vi "Ring_buffer_reader_Core.vi"() -> ()   [LabVIEW 2011]
panel:
  out "Array 2":T1(array[cluster])
  in  "Array":path[](array[path])=[path "C:/Franjo/Work/2014/CoDiS_Core/CoDiS-DM_PS_Wivenhoe/Temp/Running_Log_7/CPU_Usage (%).bin"]
  out "Remainder2":i64
  out "Loop Count 2":i32
  out "Remainder1":i64
  out "size (in bytes)":i64
  out "Loop Count 1":i32
  out "pointer":i64
  out "XY Graph":T1(graph)
  out "error out":errorcluster
  # "03:02:50"
  # "Remainder1 and Remainder2 should be zero, otherwise file is corrupted."
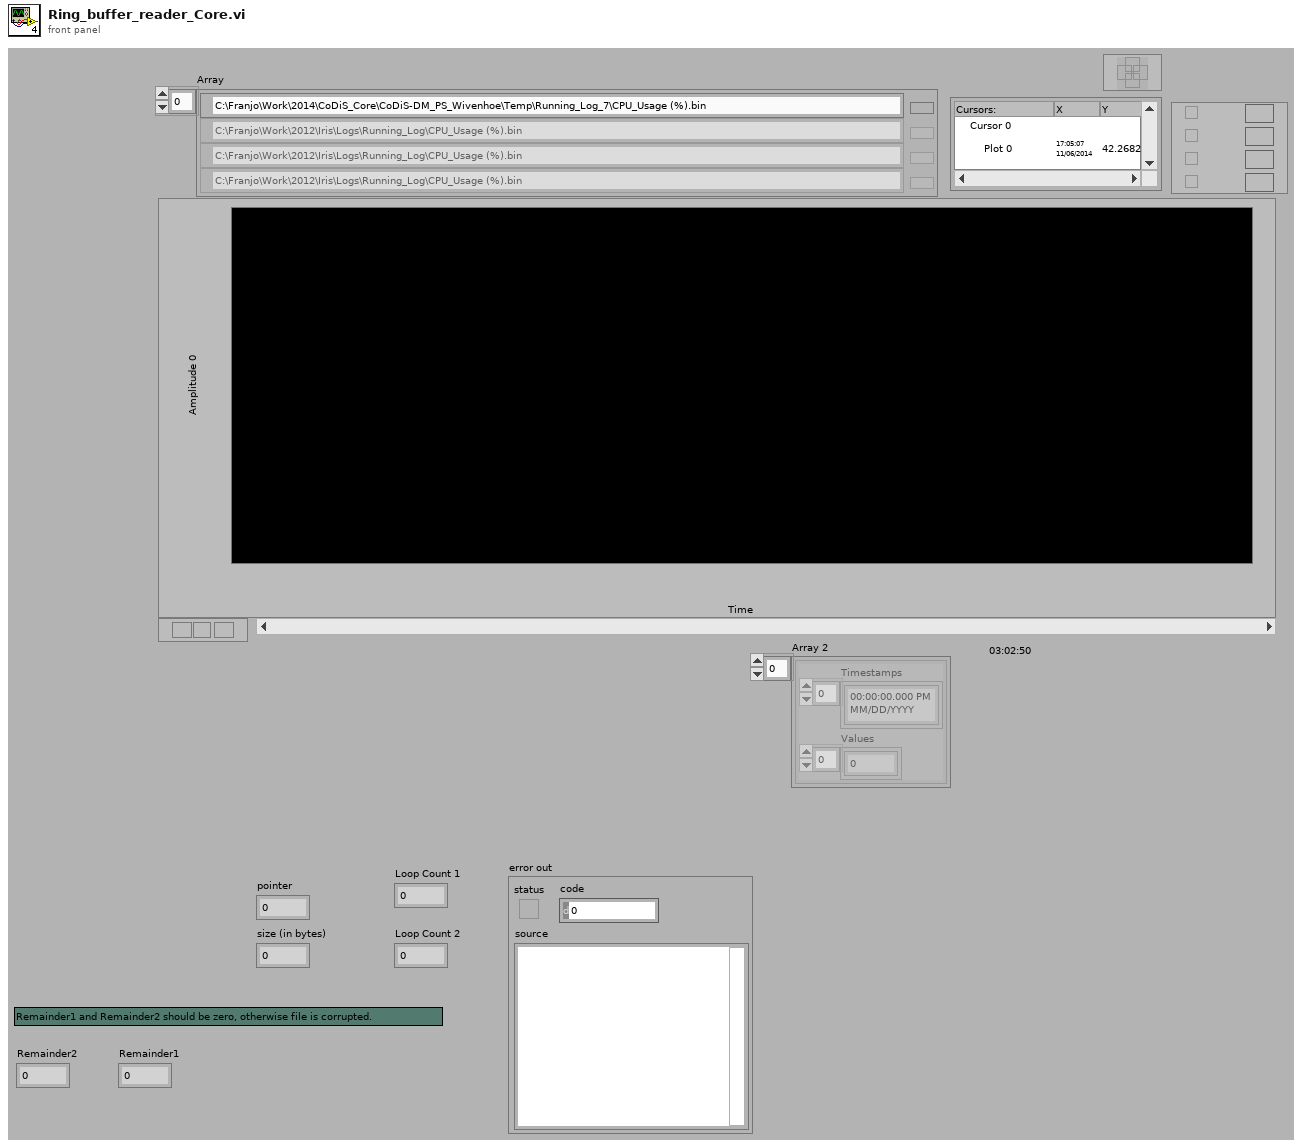
[diagram p1: front panel]
types:
  T1 = cluster{"Timestamps":timestamp[], "Values":sgl[]}[]
  T2 = cluster{"Timestamps":timestamp[], "Values":sgl[]}
  T3 = enum16{"open", "replace", "create", "open or create", "replace or create", "replace or create with confirmation"}
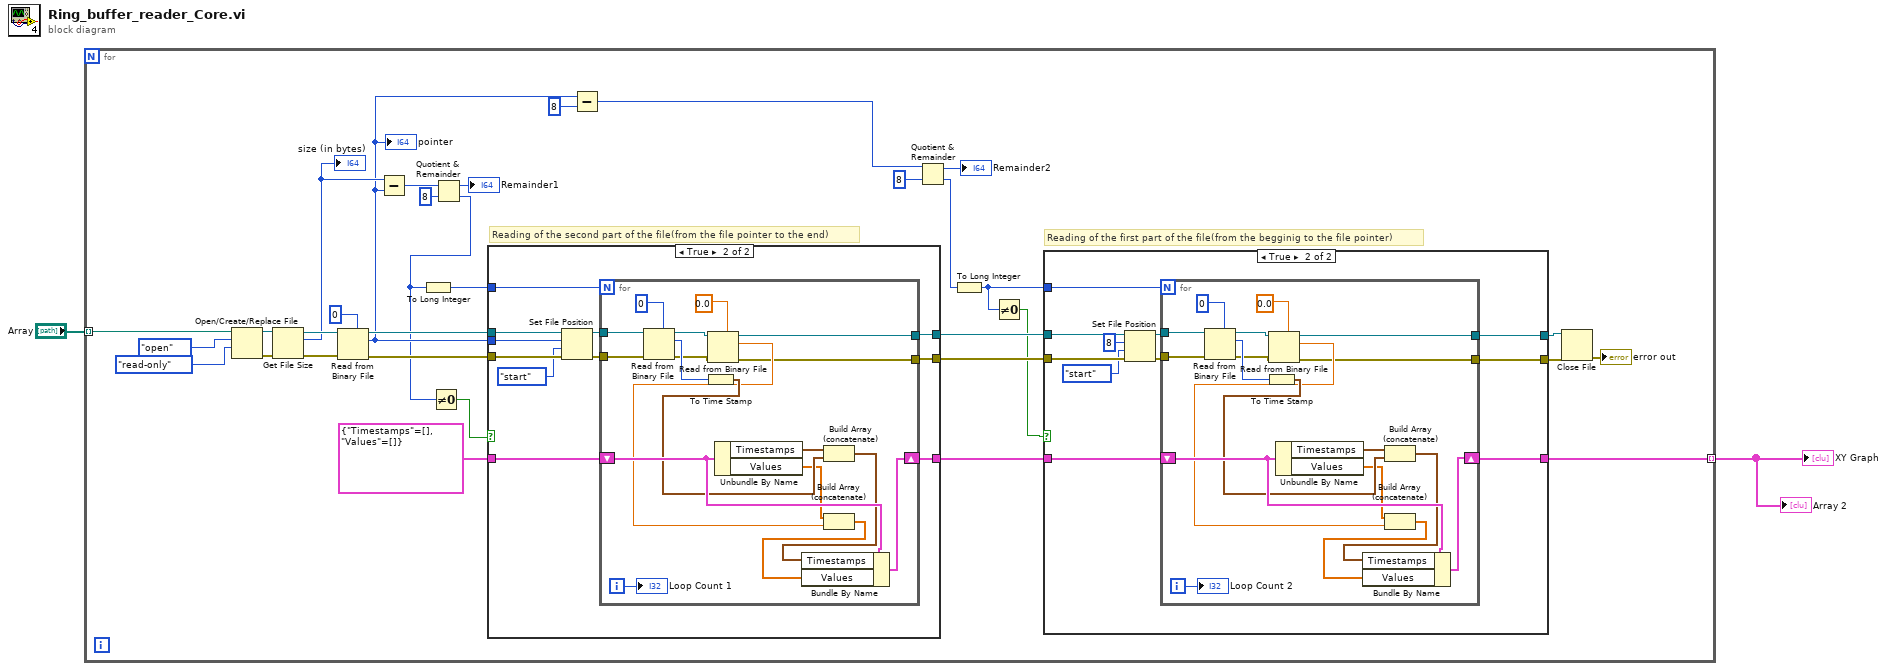
[diagram p0: block diagram]
diagram:
  n1 = for {
    tunnel: [w8] -> w1 mode=indexing
    tunnel: "Array" -> [w7] mode=indexing
    # "Reading of the second part of the file(from the file pointer to the end)"
    # "Reading of the first part of the file(from the begginig to the file pointer)"
    n2 = Open/Create/Replace File(file path (use dialog)=w7, operation (0:open)=T3."open", access (0:read/write)=enum16{"read/write", "read-only", "write-only"}."read-only") -> (refnum out=w28:refnum<file>, error out=w27:errorcluster)  [unwired: 3 in, 1 out]
    n3 = Get File Size(file=w28, error in=w27) -> (refnum out=w25:refnum<file>, size (in bytes)=w21:i64, 0:w26:errorcluster)
    "size (in bytes)" <- w21
    n4 = Read from Binary File(5:i64 0, 8:w26, 11:w25) -> (0:w30:errorcluster, 2:w14:i64, 3:w31:refnum<file>)  [unwired: 3 in, 1 out]
    "pointer" <- w14
    n5 = Subtract(x=w21, y=w14) -> (x-y=w24:i64)
    n6 = Quotient & Remainder(x=w24, y=i64 8) -> (x-y*floor(x/y)=→"Remainder1":i64, floor(x/y)=w3:i64)
    n7 = To Long Integer(number=w3) -> (32bit integer=w20:i32)
    n8 = Not Equal To 0?(x=w3) -> (x != 0?=w4:bool)
    n9 = case shown="True" w4 {
      tunnel: w31 -> [w36 w49]
      tunnel: w30 -> [w37 w48]
      tunnel: T2 {"Timestamps"=[], "Values"=[]} ("Cluster") -> [w38 w44]
      tunnel: w20 -> [_ w43]
      tunnel: [w38 w42] -> w19
      tunnel: [w37 w41] -> w18
      tunnel: [w36 w40] -> w17
      tunnel: w14 -> [_ w39]
      frame False {
      }
      frame True {
        n10 = Set File Position(offset (in bytes) (0)=w39, refnum=w49, from (0:start)=enum16{"start", "end", "current"}."start", error in=w48) -> (refnum out=w46:refnum<file>, error out=w45:errorcluster)
        n11 = for {
          N: w43 -> [_]
          tunnel: w45 -> [w66]
          tunnel: w46 -> [w67]
          tunnel: [w55] -> w40
          tunnel: [w54] -> w41
          shift-right: [w57] -> w42
          shift-left: w44 -> [w60]
          i -> [w56]
          n12 = Read from Binary File(5:u32 0, 8:w66, 11:w67) -> (0:w61:errorcluster, 2:w62:u32, 3:w64:refnum<file>)  [unwired: 3 in, 1 out]
          n13 = To Time Stamp(1:w62) -> (0:w59:timestamp)
          n14 = Read from Binary File(5:sgl 0.0, 8:w61, 11:w64) -> (0:w54:errorcluster, 2:w58:sgl, 3:w55:refnum<file>)  [unwired: 3 in, 1 out]
          n15 = Unbundle By Name(w60) -> ("Timestamps"=w53:timestamp[], "Values"=w52:sgl[])
          n16 = Build Array (concatenate)(w53, w59) -> (w50:timestamp[])
          n17 = Build Array (concatenate)(w52, w58) -> (w51:sgl[])
          n18 = Bundle By Name(cluster=w60, "Timestamps"=w50, "Values"=w51) -> (w57:T2)
          "Loop Count 1" <- w56
        }
      }
    }
    n19 = Subtract(x=w14, y=i64 8) -> (x-y=w15:i64)
    n20 = Quotient & Remainder(x=w15, y=i64 8) -> (x-y*floor(x/y)=→"Remainder2":i64, floor(x/y)=w11:i64)
    n21 = To Long Integer(number=w11) -> (32bit integer=w5:i32)
    n22 = Not Equal To 0?(x=w5) -> (x != 0?=w6:bool)
    n23 = case shown="True" w6 {
      tunnel: w19 -> [w68 w81]
      tunnel: w18 -> [w69 w78]
      tunnel: w17 -> [w70 w77]
      tunnel: [w70 w74] -> w10
      tunnel: [w69 w73] -> w9
      tunnel: [w68 w72] -> w8
      tunnel: w5 -> [_ w71]
      frame False {
      }
      frame True {
        n24 = Set File Position(offset (in bytes) (0)=i64 8, refnum=w77, from (0:start)=enum16{"start", "end", "current"}."start", error in=w78) -> (refnum out=w80:refnum<file>, error out=w79:errorcluster)
        n25 = for {
          N: w71 -> [_]
          tunnel: w79 -> [w98]
          tunnel: w80 -> [w99]
          tunnel: [w87] -> w74
          tunnel: [w86] -> w73
          shift-right: [w89] -> w72
          shift-left: w81 -> [w92]
          i -> [w88]
          n26 = Read from Binary File(5:u32 0, 8:w98, 11:w99) -> (0:w93:errorcluster, 2:w94:u32, 3:w96:refnum<file>)  [unwired: 3 in, 1 out]
          n27 = To Time Stamp(1:w94) -> (0:w91:timestamp)
          n28 = Read from Binary File(5:sgl 0.0, 8:w93, 11:w96) -> (0:w86:errorcluster, 2:w90:sgl, 3:w87:refnum<file>)  [unwired: 3 in, 1 out]
          n29 = Unbundle By Name(w92) -> ("Timestamps"=w85:timestamp[], "Values"=w84:sgl[])
          n30 = Build Array (concatenate)(w85, w91) -> (w82:timestamp[])
          n31 = Build Array (concatenate)(w84, w90) -> (w83:sgl[])
          n32 = Bundle By Name(cluster=w92, "Timestamps"=w82, "Values"=w83) -> (w89:T2)
          "Loop Count 2" <- w88
        }
      }
    }
    n33 = Close File(refnum=w10, error in=w9) -> (error out=→"error out":errorcluster)  [unwired: 1 out]
  }
  "XY Graph" <- w1
  "Array 2" <- w1
